vi "Calculate Placing Accuracy.vi"() -> ()   [LabVIEW 2017]
uses:
  Shared Components/Gantry Class/Type Definitions/Virtual Modes.ctl
  Shared Components/Gantry Class/Type Definitions/Init_Modes.ctl
  Shared Components/Config Manager Class/Type Definitions/Camera Enum.ctl
  Shared Components/Gantry Class/Gantry Class.lvclass
  Shared Components/Vec3d Class/Vec3d Class.lvclass
panel:
  out "Iteration Number":i32
  out "Point being recorded":string="\\P"
  in  "Results Folder":path=path "C:/Users/Admin/Gantry Purdue/pixel-gantry-control/Config"
  in  "Virtual Mode":T1=enum."Virtual"
  in  "stop":bool
  out "Image":T2(plugin-control)
  out "error out":errorcluster
  in  "Config Folder":path=path "C:/Users/Admin/Gantry Purdue/pixel-gantry-control/Config"
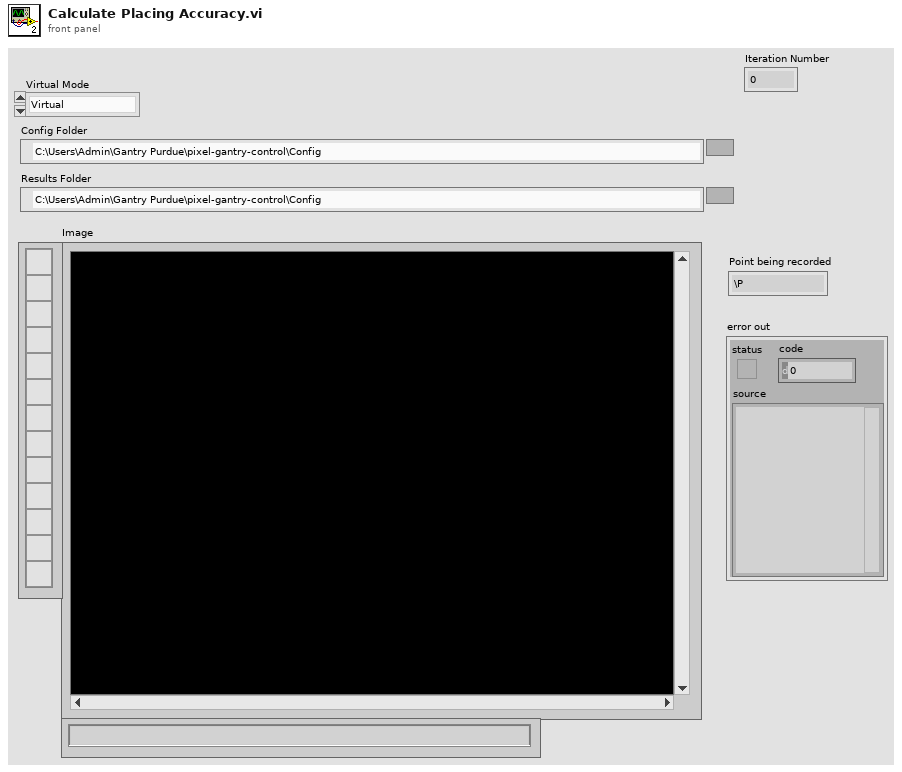
[diagram p1: front panel]
types:
  T1 = typedef "Virtual Modes.ctl" = enum16{"Nonvirtual", "Pseudovirtual", "Virtual"}
  T2 = typedef "IMAQ Image.ctl" = refnum<image>
  T3 = typedef "Init_Modes.ctl" = enum16{"Full", "Robot Only", "Dispenser Only", "Cameras Only", "Robot and Cameras", "Robot and Cameras and Dispenser", "Manifold Only"}
  T4 = typedef "Camera Enum.ctl" = enum16{"GANTRY HEAD", "NEEDLE CALIBRATION X", "NEEDLE CALIBRATION Y", "STAND CAMERA", "SIMRAN WEBCAM"}
  T5 = typedef "Physical Image.ctl" = cluster{"Image Position":refnum<class "Vec3d Class.lvclass">, "Image Reference":T2, "Field of View":cluster{"x(mm)":dbl, "y(mm)":dbl}}
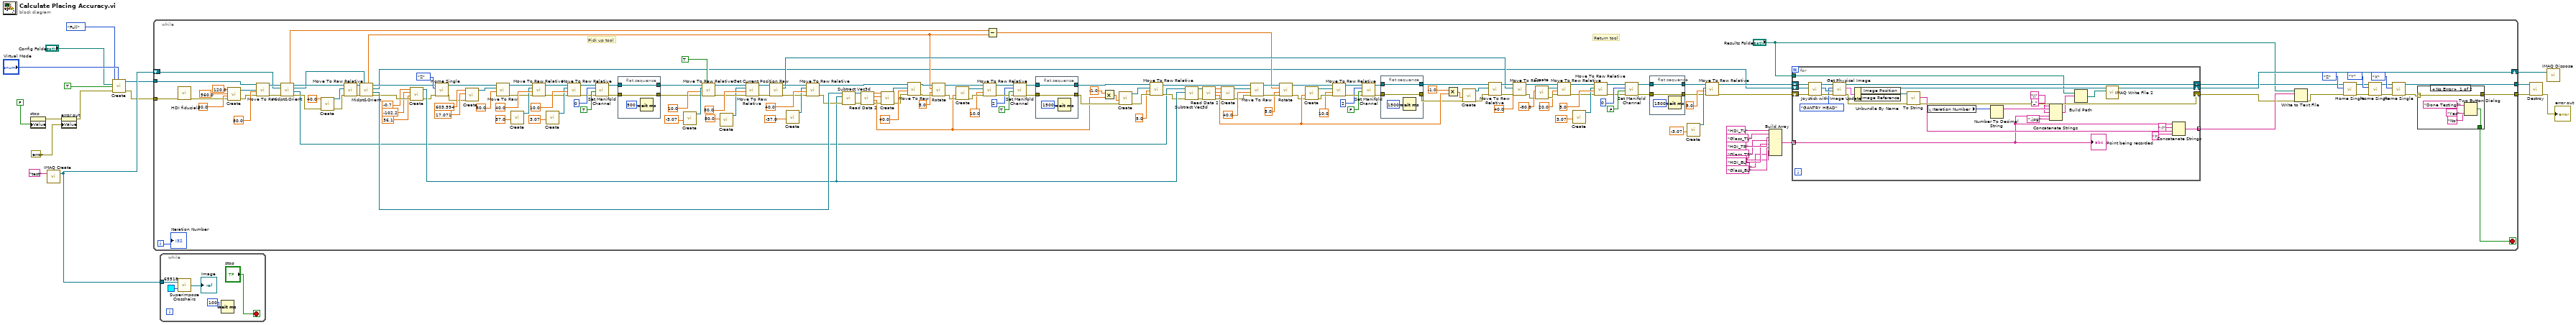
[diagram p0: block diagram]
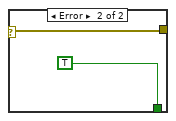
[diagram p2: hidden frame]
diagram:
  n1 = property on="stop" class="Bool (strict)"("Value"=FALSE) -> (error out=w14:errorcluster)  [unwired: 2 in, 1 out]
  n2 = call "IMAQ Create"("Image Name"="test") -> ("New Image"=w11:T2)  [unwired: 4 in, 1 out]
  n3 = property on="error out" class="Clust (strict)"(error in=w14, "Value"=errorcluster {"status"=FALSE, "code"=0, "source"=""} ("error in (no error)")) -> (error out=w6:errorcluster)  [unwired: 1 in, 1 out]
  n4 = call "Create.vi"("Virtual Mode"="Virtual Mode", "error in"=w6, "HOME?"=TRUE, "Config Folder"="Config Folder", "Init Mode"=Init_Modes."Full") -> ("error out"=w3:errorcluster, "Gantry out"=w2:refnum<class "Gantry Class.lvclass">)  [unwired: 5 in]
  n5 = while {
    tunnel: [w64] -> w9
    tunnel: [w37] -> w8
    shift-right: [w31] -> w10
    shift-left: w11 -> [w144]
    tunnel: w3 -> [w40]
    tunnel: w2 -> [w39]
    i -> [w17]
    stop <- w36 stop-if-true
    # "Pick up tool"
    # "Return tool"
    n6 = call "HDI fiducials"("error in (no error)"=w40) -> ("error out"=w60:errorcluster)  [unwired: 17 in, 1 out]
    n7 = call "Create.vi"("error in"=w60, "Z"=30.0, "Y"=560.0, "X"=120.0) -> ("error out"=w150:errorcluster, "Vec3d Class out"=w185:refnum<class "Vec3d Class.lvclass">)  [unwired: 6 in]
    n8 = call-dynamic "Move To Raw.vi"("error in"=w150, "Speed"=80.0, "Destination"=w185, "Gantry in"=w39) -> ("error out"=w149:errorcluster, "Gantry out"=w148:refnum<class "Gantry Class.lvclass">)  [unwired: 6 in]
    n9 = call-dynamic "Midpt&Orient.vi"("error in (no error)"=w149, "Image In"=w144, "Gantry Class in"=w148) -> ("error out"=w57:errorcluster, "Midpoint"=w51:refnum<class "Vec3d Class.lvclass">, "Image Out"=w143:T2, "Gantry Class out"=w147:refnum<class "Gantry Class.lvclass">, "Orientation"=w42:dbl)  [unwired: 4 in]
    n10 = call "Create.vi"("error in"=w57, "X"=40.0) -> ("error out"=w58:errorcluster, "Vec3d Class out"=w59:refnum<class "Vec3d Class.lvclass">)  [unwired: 8 in]
    n11 = call-dynamic "Move To Raw Relative.vi"("error in"=w58, "Delta"=w59, "Gantry in"=w147) -> ("error out"=w146:errorcluster, "Gantry out"=w145:refnum<class "Gantry Class.lvclass">)  [unwired: 7 in]
    n12 = call-dynamic "Midpt&Orient.vi"("error in (no error)"=w146, "Image In"=w143, "Gantry Class in"=w145) -> ("error out"=w55:errorcluster, "Midpoint"=w141:refnum<class "Vec3d Class.lvclass">, "Image Out"=w32:T2, "Gantry Class out"=w46:refnum<class "Gantry Class.lvclass">, "Orientation"=w43:dbl)  [unwired: 4 in]
    n13 = call "Create.vi"("error in"=w55, "Z"=36.1 ("Y"), "Y"=-102.2, "X"=-0.7) -> ("error out"=w47:errorcluster, "Vec3d Class out"=w104:refnum<class "Vec3d Class.lvclass">)  [unwired: 6 in]
    n14 = call-dynamic "Home Single.vi"("error in"=w47, "Axis"=enum16{"X", "Y", "Z", "U"}."Z", "Gantry in"=w46) -> ("error out"=w44:errorcluster, "Gantry out"=w45:refnum<class "Gantry Class.lvclass">)  [unwired: 7 in]
    n15 = call "Create.vi"("error in"=w44, "Y"=17.071, "X"=603.594) -> ("Vec3d Class out"=w206:refnum<class "Vec3d Class.lvclass">)  [unwired: 7 in, 1 out]
    n16 = call-dynamic "Move To Raw.vi"("Speed"=80.0 ("Speed(mm/s)"), "Destination"=w206, "Gantry in"=w45) -> ("error out"=w73:errorcluster, "Gantry out"=w75:refnum<class "Gantry Class.lvclass">)  [unwired: 7 in]
    n17 = call "Create.vi"("Z"=37.0) -> ("Vec3d Class out"=w76:refnum<class "Vec3d Class.lvclass">)  [unwired: 9 in, 1 out]
    n18 = call-dynamic "Move To Raw Relative.vi"("error in"=w73, "Speed(mm/s)"=40.0, "Delta"=w76, "Gantry in"=w75) -> ("Gantry out"=w74:refnum<class "Gantry Class.lvclass">)  [unwired: 6 in, 1 out]
    n19 = call "Create.vi"("Z"=3.07) -> ("Vec3d Class out"=w200:refnum<class "Vec3d Class.lvclass">)  [unwired: 9 in, 1 out]
    n20 = call-dynamic "Move To Raw Relative.vi"("error in"=w73, "Speed(mm/s)"=10.0, "Delta"=w200, "Gantry in"=w74) -> ("error out"=w198:errorcluster, "Gantry out"=w199:refnum<class "Gantry Class.lvclass">)  [unwired: 6 in]
    n21 = call-dynamic "Set Manifold Channel.vi"("error in"=w198, "On/Off"=TRUE, "Manifold Channel"=0, "Gantry in"=w199) -> ("error out"=w157:errorcluster, "Gantry out"=w159:refnum<class "Gantry Class.lvclass">)  [unwired: 6 in]
    n22 = flat-sequence {
      tunnel: w159 -> [w253]
      tunnel: [w253] -> w158
      tunnel: w157 -> [w251]
      tunnel: [w251] -> w156
      frame #0 {
        n23 = Wait (ms)(milliseconds to wait=u32 500) -> ()  [unwired: 1 out]
      }
    }
    n24 = call "Create.vi"("Z"=-3.07) -> ("Vec3d Class out"=w196:refnum<class "Vec3d Class.lvclass">)  [unwired: 9 in, 1 out]
    n25 = call-dynamic "Move To Raw Relative.vi"("Wait?"=TRUE, "error in"=w156, "Speed(mm/s)"=10.0, "Delta"=w196, "Gantry in"=w158) -> ("error out"=w191:errorcluster, "Gantry out"=w192:refnum<class "Gantry Class.lvclass">)  [unwired: 5 in]
    n26 = call "Create.vi"("Y"=80.0 ("Z")) -> ("Vec3d Class out"=w190:refnum<class "Vec3d Class.lvclass">)  [unwired: 9 in, 1 out]
    n27 = call-dynamic "Move To Raw Relative.vi"("error in"=w191, "Speed(mm/s)"=80.0, "Delta"=w190, "Gantry in"=w192) -> ("error out"=w178:errorcluster, "Gantry out"=w180:refnum<class "Gantry Class.lvclass">)  [unwired: 6 in]
    n28 = call-dynamic "Get Current Position Raw.vi"("error in"=w178, "Gantry in"=w180) -> ("error out"=w177:errorcluster, "Vec3d Class out"=w92:refnum<class "Vec3d Class.lvclass">, "Gantry out"=w179:refnum<class "Gantry Class.lvclass">)  [unwired: 7 in]
    n29 = call "Create.vi"("Z"=-37.0) -> ("Vec3d Class out"=w186:refnum<class "Vec3d Class.lvclass">)  [unwired: 9 in, 1 out]
    n30 = call-dynamic "Move To Raw Relative.vi"("error in"=w177, "Speed(mm/s)"=40.0, "Delta"=w186, "Gantry in"=w179) -> ("error out"=w135:errorcluster, "Gantry out"=w133:refnum<class "Gantry Class.lvclass">)  [unwired: 6 in]
    n31 = call "Subtract Vec3d.vi"("error in (no error)"=w135, "Vec3d in 2"=w104, "Vec3d in 1"=w141) -> ("error out"=w137:errorcluster, "Vec3d Class out"=w80:refnum<class "Vec3d Class.lvclass">)  [unwired: 7 in]
    n32 = call-dynamic "Read Data 2.vi"("error in"=w137, "Vec3d in"=w80) -> ("error out"=w136:errorcluster, "Z"=w81:dbl, "Y"=w139:dbl, "X"=w140:dbl)  [unwired: 6 in]
    n33 = call "Create.vi"("error in"=w136, "Y"=w139, "X"=w140) -> ("error out"=w134:errorcluster, "Vec3d Class out"=w79:refnum<class "Vec3d Class.lvclass">)  [unwired: 7 in]
    n34 = call-dynamic "Move To Raw.vi"("error in"=w134, "Speed"=40.0, "Destination"=w79, "Gantry in"=w133) -> ("error out"=w91:errorcluster, "Gantry out"=w90:refnum<class "Gantry Class.lvclass">)  [unwired: 6 in]
    n35 = call-dynamic "Rotate.vi"("error in"=w91, "speed(deg/s)"=5.0, "distance(deg)"=w43, "Gantry in"=w90) -> ("error out"=w88:errorcluster, "Gantry out"=w89:refnum<class "Gantry Class.lvclass">)  [unwired: 6 in]
    n36 = call "Create.vi"("error in"=w88, "Z"=w81) -> ("error out"=w132:errorcluster, "Vec3d Class out"=w138:refnum<class "Vec3d Class.lvclass">)  [unwired: 8 in]
    n37 = call-dynamic "Move To Raw Relative.vi"("error in"=w132, "Speed(mm/s)"=10.0, "Delta"=w138, "Gantry in"=w89) -> ("error out"=w126:errorcluster, "Gantry out"=w127:refnum<class "Gantry Class.lvclass">)  [unwired: 6 in]
    n38 = Subtract(x=w42, y=w43) -> (x-y=w41:dbl)
    n39 = call-dynamic "Set Manifold Channel.vi"("error in"=w126, "On/Off"=TRUE, "Manifold Channel"=2, "Gantry in"=w127) -> ("error out"=w128:errorcluster, "Gantry out"=w129:refnum<class "Gantry Class.lvclass">)  [unwired: 6 in]
    n40 = flat-sequence {
      tunnel: w129 -> [w247]
      tunnel: [w247] -> w124
      tunnel: w128 -> [w245]
      tunnel: [w245] -> w123
      frame #0 {
        n41 = Wait (ms)(milliseconds to wait=u32 1500) -> ()  [unwired: 1 out]
      }
    }
    n42 = Multiply(x=-1.0, y=w81) -> (x*y=w183:dbl)
    n43 = call "Create.vi"("error in"=w123, "Z"=w183) -> ("error out"=w181:errorcluster, "Vec3d Class out"=w182:refnum<class "Vec3d Class.lvclass">)  [unwired: 8 in]
    n44 = call-dynamic "Move To Raw Relative.vi"("error in"=w181, "Speed(mm/s)"=5.0, "Delta"=w182, "Gantry in"=w124) -> ("error out"=w98:errorcluster, "Gantry out"=w99:refnum<class "Gantry Class.lvclass">)  [unwired: 6 in]
    n45 = call "Subtract Vec3d.vi"("error in (no error)"=w98, "Vec3d in 2"=w104, "Vec3d in 1"=w51) -> ("error out"=w113:errorcluster, "Vec3d Class out"=w116:refnum<class "Vec3d Class.lvclass">)  [unwired: 7 in]
    n46 = call-dynamic "Read Data 2.vi"("error in"=w113, "Vec3d in"=w116) -> ("error out"=w112:errorcluster, "Z"=w103:dbl, "Y"=w117:dbl, "X"=w118:dbl)  [unwired: 6 in]
    n47 = call "Create.vi"("error in"=w112, "Y"=w117, "X"=w118) -> ("error out"=w111:errorcluster, "Vec3d Class out"=w115:refnum<class "Vec3d Class.lvclass">)  [unwired: 7 in]
    n48 = call-dynamic "Move To Raw.vi"("error in"=w111, "Speed"=40.0, "Destination"=w115, "Gantry in"=w99) -> ("error out"=w85:errorcluster, "Gantry out"=w86:refnum<class "Gantry Class.lvclass">)  [unwired: 6 in]
    n49 = call-dynamic "Rotate.vi"("error in"=w85, "speed(deg/s)"=5.0, "distance(deg)"=w41, "Gantry in"=w86) -> ("error out"=w84:errorcluster, "Gantry out"=w83:refnum<class "Gantry Class.lvclass">)  [unwired: 6 in]
    n50 = call "Create.vi"("error in"=w84, "Z"=w103) -> ("error out"=w110:errorcluster, "Vec3d Class out"=w114:refnum<class "Vec3d Class.lvclass">)  [unwired: 8 in]
    n51 = call-dynamic "Move To Raw Relative.vi"("error in"=w110, "Speed(mm/s)"=10.0, "Delta"=w114, "Gantry in"=w83) -> ("error out"=w106:errorcluster, "Gantry out"=w107:refnum<class "Gantry Class.lvclass">)  [unwired: 6 in]
    n52 = call-dynamic "Set Manifold Channel.vi"("error in"=w106, "On/Off"=FALSE, "Manifold Channel"=2, "Gantry in"=w107) -> ("error out"=w102:errorcluster, "Gantry out"=w100:refnum<class "Gantry Class.lvclass">)  [unwired: 6 in]
    n53 = flat-sequence {
      tunnel: w100 -> [w244]
      tunnel: [w244] -> w96
      tunnel: w102 -> [w242]
      tunnel: [w242] -> w101
      frame #0 {
        n54 = Wait (ms)(milliseconds to wait=u32 1500) -> ()  [unwired: 1 out]
      }
    }
    n55 = Multiply(x=-1.0, y=w103) -> (x*y=w120:dbl)
    n56 = call "Create.vi"("error in"=w101, "Z"=w120) -> ("error out"=w97:errorcluster, "Vec3d Class out"=w93:refnum<class "Vec3d Class.lvclass">)  [unwired: 8 in]
    n57 = call-dynamic "Move To Raw Relative.vi"("error in"=w97, "Delta"=w93, "Gantry in"=w96) -> ("error out"=w94:errorcluster, "Gantry out"=w95:refnum<class "Gantry Class.lvclass">)  [unwired: 7 in]
    n58 = call-dynamic "Move To Raw.vi"("error in"=w94, "Speed"=40.0, "Destination"=w92, "Gantry in"=w95) -> ("error out"=w63:errorcluster, "Gantry out"=w72:refnum<class "Gantry Class.lvclass">)  [unwired: 6 in]
    n59 = call "Create.vi"("error in"=w63, "Y"=-80.0) -> ("error out"=w175:errorcluster, "Vec3d Class out"=w160:refnum<class "Vec3d Class.lvclass">)  [unwired: 8 in]
    n60 = call-dynamic "Move To Raw Relative.vi"("error in"=w175, "Speed(mm/s)"=20.0, "Delta"=w160, "Gantry in"=w72) -> ("error out"=w161:errorcluster, "Gantry out"=w162:refnum<class "Gantry Class.lvclass">)  [unwired: 6 in]
    n61 = call "Create.vi"("Z"=3.07) -> ("Vec3d Class out"=w168:refnum<class "Vec3d Class.lvclass">)  [unwired: 9 in, 1 out]
    n62 = call-dynamic "Move To Raw Relative.vi"("error in"=w161, "Speed(mm/s)"=5.0, "Delta"=w168, "Gantry in"=w162) -> ("error out"=w166:errorcluster, "Gantry out"=w167:refnum<class "Gantry Class.lvclass">)  [unwired: 6 in]
    n63 = call-dynamic "Set Manifold Channel.vi"("error in"=w166, "On/Off"=FALSE, "Manifold Channel"=0, "Gantry in"=w167) -> ("error out"=w153:errorcluster, "Gantry out"=w155:refnum<class "Gantry Class.lvclass">)  [unwired: 6 in]
    n64 = flat-sequence {
      tunnel: w155 -> [w250]
      tunnel: [w250] -> w154
      tunnel: w153 -> [w248]
      tunnel: [w248] -> w152
      frame #0 {
        n65 = Wait (ms)(milliseconds to wait=u32 1500) -> ()  [unwired: 1 out]
      }
    }
    n66 = call "Create.vi"("Z"=-3.07) -> ("Vec3d Class out"=w164:refnum<class "Vec3d Class.lvclass">)  [unwired: 9 in, 1 out]
    n67 = call-dynamic "Move To Raw Relative.vi"("error in"=w152, "Speed(mm/s)"=5.0, "Delta"=w164, "Gantry in"=w154) -> ("error out"=w35:errorcluster, "Gantry out"=w34:refnum<class "Gantry Class.lvclass">)  [unwired: 6 in]
    n68 = Build Array("HDI_TL" ("string"), "Glass_TL" ("string"), "HDI_TR" ("string"), "Glass_TR" ("string"), "HDI_BL" ("string"), "Glass_BL" ("string"), "HDI_BR" ("string"), "Glass_BR" ("string")) -> (w21:string[])
    n69 = for {
      tunnel: [w224] -> w33 mode=indexing
      shift-right: [w225] -> w19
      shift-left: w35 -> [w228]
      shift-right: [w223] -> w30
      shift-left: w34 -> [w227]
      shift-right: [w212] -> w31
      shift-left: w32 -> [w222]
      tunnel: w21 -> [w214] mode=indexing
      tunnel: "Results Folder" -> [w215]
      n70 = call-dynamic "Joystick with Image Update.vi"("error in (no error)"=w228, "Image In"=w222, "Gantry Class in"=w227) -> ("error out"=w234:errorcluster, "Image Out"=w221:T2, "Gantry Class out"=w233:refnum<class "Gantry Class.lvclass">)  [unwired: 6 in]
      n71 = call-dynamic "Get Physical Image.vi"("error in"=w234, "Image In"=w221, "Camera Name"=Camera_Enum."GANTRY HEAD", "Gantry in"=w233) -> ("error out"=w226:errorcluster, "Physical Image"=w232:T5, "Gantry out"=w223:refnum<class "Gantry Class.lvclass">)  [unwired: 5 in]
      n72 = Unbundle By Name(w232) -> ("Image Position"=w231:refnum<class "Vec3d Class.lvclass">, "Image Reference"=w219:T2)
      n73 = call "To String.vi"("error in"=w226, "Vec3d in"=w231) -> ("error out"=w225:errorcluster, "Vec3d String"=w229:string)  [unwired: 7 in, 1 out]
      n74 = local read "Iteration Number"() -> (w211:i32)
      n75 = Number To Decimal String(number=w211) -> (decimal integer string=w209:string)  [unwired: 1 in]
      n76 = Concatenate Strings("\\" ("string"), w209, "_" ("string"), w214, ".jpg" ("string")) -> (w217:string)
      n77 = Build Path(base path=w215, name or relative path=w217) -> (appended path=w218:path)
      n78 = call-poly "IMAQ Write File 2"("File Path"=w218, "Image"=w219) -> ("Image Out (duplicate)"=w212:T2)  [unwired: 8 in, 1 out]
      n79 = Concatenate Strings(w214, ":(" ("string"), w229, ")" ("string")) -> (w224:string)
      "Point being recorded" <- w214
    }
    n80 = Write to Text File(file (use dialog)="Results Folder", text=w33, error in=w19) -> (error out=w18:errorcluster)  [unwired: 1 in, 2 out]
    n81 = call-dynamic "Home Single.vi"("error in"=w18, "Axis"=enum16{"X", "Y", "Z", "U"}."Z", "Gantry in"=w30) -> ("error out"=w67:errorcluster, "Gantry out"=w68:refnum<class "Gantry Class.lvclass">)  [unwired: 7 in]
    n82 = call-dynamic "Home Single.vi"("error in"=w67, "Axis"=enum16{"X", "Y", "Z", "U"}."Y", "Gantry in"=w68) -> ("error out"=w65:errorcluster, "Gantry out"=w66:refnum<class "Gantry Class.lvclass">)  [unwired: 7 in]
    n83 = call-dynamic "Home Single.vi"("error in"=w65, "Axis"=enum16{"X", "Y", "Z", "U"}."X", "Gantry in"=w66) -> ("error out"=w38:errorcluster, "Gantry out"=w64:refnum<class "Gantry Class.lvclass">)  [unwired: 7 in]
    n84 = case shown="No Error" w38 {
      selector: w38 -> [w235 w241]
      tunnel: [w235 w241] -> w37
      tunnel: [w236 TRUE ("Done Testing?")] -> w36
      frame No Error {
        n85 = Two Button Dialog(message="Done Testing?", 1:"No" ("F button name (\"Cancel\")"), 2:"Yes" ("T button name (\"OK\")")) -> (T button?=w236:bool)
      }
      frame Error {
      }
    }
    "Iteration Number" <- w17
  }
  n86 = while {
    tunnel: w11 -> [w256]
    stop <- "stop" stop-if-true
    n87 = call "Superimpose Crosshairs.vi"("Grid Line Color"=u32 65518, "Refnum in"=w256) -> ("Refnum out"=→"Image":T2)
    n88 = Wait (ms)(milliseconds to wait=u32 100) -> ()  [unwired: 1 out]
  }
  n89 = call "Destroy.vi"("error in"=w8, "Gantry Class in"=w9) -> ("error out"=→"error out":errorcluster)  [unwired: 9 in]
  n90 = call "IMAQ Dispose"("Image"=w10) -> ()  [unwired: 5 in, 1 out]
